vi "Get Estimate Time.vi"(9 "Speed":i32, 10 "Current SP":dbl, 11 "Next SP":dbl) -> (3 "time stamp":timestamp)   [LabVIEW 2020]
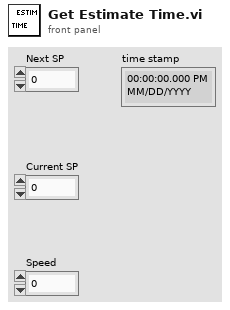
[diagram p1: front panel]
types:
  T1 = typedef "LVDateTimeRec.ctl" = cluster{"fractional second":dbl, "second":i32, "minute":i32, "hour":i32, "day of month":i32, "month":i32, "year":i32, "day of week":i32, "day of year":i32, "DST":i32}
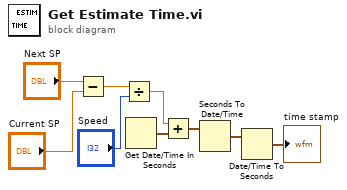
[diagram p0: block diagram]
diagram:
  n1 = Subtract(x="Next SP", y="Current SP") -> (x-y=w1:dbl)
  n2 = Divide(x=w1, y="Speed") -> (x/y=w9:dbl)
  n3 = Get Date/Time In Seconds() -> (seconds since 1Jan1904=w6:timestamp)
  n4 = Add(x=w9, y=w6) -> (x+y=w8:timestamp)
  n5 = Seconds To Date/Time(time stamp (now)=w8) -> (date time rec=w7:T1)  [unwired: 1 in]
  n6 = Date/Time To Seconds(2:w7) -> (0:→"time stamp":timestamp)  [unwired: 1 in]
